vi "SigSyn (G3)-Compute Max Level.vi"(0 "Waveform In":T1, 1 "Destination":string, 5 "Filter":T22 {"Stages"."IIR Filter"."Forward Coefficients" format="%.4f"; "Stages"."IIR Filter"."Reverse Coefficients" format="%.4f"}, 9 "Level":T20, 11 "error in (no error)":errorcluster, 12 "Sampling Rate (Hz)":dbl, 13 "Npts":i32) -> (4 "Waveform Out":T1={"Type"=enum."Tone", "Tone"={"Frequency (kHz)"=0.0, "Phase (cycles)"=0.0, "Random phase"=FALSE}, "Pulse Train"={"Pulse width (us)"=0.0, "Pulse rate (Hz)"=0.0, "Gap (ms)"=0.0, "Polarity"=enum."POS", "PT State"={"Template"=[], "Nperiod"=0, "Index"=0, "Pulse Rate (Hz)"=0.0, "Phase (cycles)"=0.0, "Noff"=0}, "Asynch"=FALSE}, "Noise"={"Properties"={"InvFilt"=FALSE, "Aweight"=FALSE, "Seed"=0, "Tokens"=0, "Brickwall"=FALSE}, "Data"={"TokenNum"=0}}, "File"={"Filename"=path "", "Signal"=[], "Channel"=0, "stream"=FALSE, "offset"=0, "nreps"=0, "loops"=0, "Randomize"=FALSE, "order"=[], "Seed"=0, "Tokens"=0}, "FMSweep"={"Rate (oct/s)"=0.0, "Fmin (Hz)"=0.0, "Fmax (Hz)"=0.0, "Ramp (ms)"=0.0, "Linear"=FALSE}, "Chirp Train"={"Params"={"Fmin (kHz)"=4.0, "Fmax (kHz)"=64.0, "Compensate"=FALSE, "Duration (ms)"=2.0}, "Data"={"WF"=[]}}, "Complex Tone"={"Params"={"F0 (Hz)"=0.0, "Band"={"Flow (Hz)"=0.0, "Fhigh (Hz)"=0.0}, "Phase"=enum."Cosine", "Min F0 (Hz)"=0.0, "Max F0 (Hz)"=0.0, "ContinRandPhase"=FALSE, "Max peak factor"=inf, "Max mod depth"=2.0, "MinHarmNum"=0, "MaxHarmNum"=0, "Level Mode"=enum."per component", "% jitter"=0.0}, "Data"={"Ncomp"=0, "MinHarm"=0, "Phase"=[], "Amplitude"=[], "Npts/frame"=0, "Last F0"=0.0, "Fmin"=0.0, "Fmax"=0.0, "Lslope"=0.0, "randphase"=FALSE, "overall rms"=FALSE, "fmult"=[], "jittered"=FALSE}}, "FM"={"Carrier (kHz)"=0.0, "ModRate (Hz)"=0.0, "Depth (Hz)"=0.0, "Phase (cycles)"=0.0}, "Vowel"={"Freqs"="", "Set level"=enum."Total", "Freq"=[], "weights"=[]}, "Ramp"={"Duration (ms)"=0.0}}, 10 "Level out":T20, 14 "Max Level":dbl, 15 "error out":errorcluster)   [LabVIEW 2020]
uses:
  XControls/Waveform XControls/Waveform (G3)/Waveform Data.ctl
  Waveform VIs/Waveform Enum (V3).ctl
  XControls/Waveform XControls/Tone (G3)/Tone.Properties.ctl
  Waveform VIs/Pulse Train VIs/Pulse Train Params.ctl
  Waveform VIs/Pulse Train VIs/Pulse Polarity.ctl
  Waveform VIs/Pulse Train VIs/PT-Continuous State.ctl
  Waveform VIs/Noise VIs/Noise (G3).ctl
  Waveform VIs/Noise VIs/Noise (G3).Properties.ctl
  Waveform VIs/Noise VIs/Noise (G3).Data.ctl
  Waveform VIs/File VIs/StimFile-Params.ctl
  Waveform VIs/FM Sweep VIs/FM Sweep Params.ctl
  Waveform VIs/Chirp Train VIs/Chirp Train.ctl
  Waveform VIs/Chirp Train VIs/Chirp Train Params.ctl
  Waveform VIs/Complex Tone VIs/CT-Params.ctl
  Waveform VIs/Complex Tone VIs/CT-Phase Enum.ctl
  Waveform VIs/Complex Tone VIs/CT-Runtime Data.ctl
  XControls/Waveform XControls/FM Tone/Data.ctl
  XControls/Waveform XControls/Vowel/Vowel.Properties.ctl
  Waveform VIs/Ramp VIs/Ramp.Properties.ctl
  XControls/Filter (G3)/Filter Data.ctl
  XControls/Filter (G3)/Filter Type.ctl
  Filter VIs/Filter-Bandwidth Units.ctl
  XControls/Level (G3)/Level Data.ctl
  XControls/Level (G3)/Level Units (G3).ctl
  XControls/Waveform XControls/Waveform (G3)/Waveform (G3).xctl
  XControls/Level (G3)/Level (G3).xctl
  XControls/Filter (G3)/Filter (G3).xctl
  XControls/Waveform XControls/Tone (G3)/Tone (G3).xctl
  XControls/Waveform XControls/FM Tone/FM Tone.xctl
  XControls/Waveform XControls/Vowel/Vowel.xctl
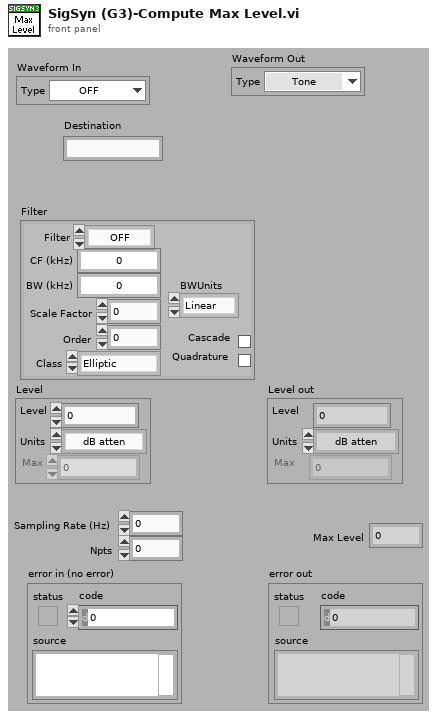
[diagram p1: front panel]
types:
  T1 = typedef "Waveform (G3).xctl/Waveform Data.ctl" = cluster{"Type":T2, "Tone":T3, "Pulse Train":T4, "Noise":T7, "File":T10, "FMSweep":T11, "Chirp Train":T12, "Complex Tone":cluster{"Params":T14, "Data":T16}, "FM":T17, "Vowel":T18, "Ramp":T19}
  T2 = typedef "Waveform Enum (V3).ctl" = enum16{"OFF", "Tone", "Noise", "Pulse Train", "File", "FM Sweep", "Chirp Train", "Complex Tone", "FM Tone", "Vowel", "Ramp"}
  T3 = typedef "Tone (G3).xctl/Tone.Properties.ctl" = cluster{"Frequency (kHz)":dbl, "Phase (cycles)":dbl, "Random phase":bool}
  T4 = typedef "Pulse Train Params.ctl" = cluster{"Pulse width (us)":dbl, "Pulse rate (Hz)":dbl, "Gap (ms)":dbl, "Polarity":T5, "PT State":T6, "Asynch":bool}
  T5 = typedef "Pulse Polarity.ctl" = enum16{"POS", "NEG", "POS-NEG", "NEG-POS"}
  T6 = typedef "PT-Continuous State.ctl" = cluster{"Template":dbl[], "Nperiod":i32, "Index":i32, "Pulse Rate (Hz)":dbl, "Phase (cycles)":dbl, "Noff":i32}
  T7 = typedef "Noise (G3).ctl" = cluster{"Properties":T8, "Data":T9}
  T8 = typedef "Noise (G3).Properties.ctl" = cluster{"InvFilt":bool, "Aweight":bool, "Seed":i32, "Tokens":i32, "Brickwall":bool}
  T9 = typedef "Noise (G3).Data.ctl" = cluster{"TokenNum":i32}
  T10 = typedef "StimFile-Params.ctl" = cluster{"Filename":path, "Signal":dbl[], "Channel":i32, "stream":bool, "offset":i32, "nreps":i32, "loops":i32, "Randomize":bool, "order":i32[], "Seed":i32, "Tokens":i32}
  T11 = typedef "FM Sweep Params.ctl" = cluster{"Rate (oct/s)":dbl, "Fmin (Hz)":dbl, "Fmax (Hz)":dbl, "Ramp (ms)":dbl, "Linear":bool}
  T12 = typedef "Chirp Train.ctl" = cluster{"Params":T13, "Data":cluster{"WF":dbl[]}}
  T13 = typedef "Chirp Train Params.ctl" = cluster{"Fmin (kHz)":dbl, "Fmax (kHz)":dbl, "Compensate":bool, "Duration (ms)":dbl}
  T14 = typedef "CT-Params.ctl" = cluster{"F0 (Hz)":dbl, "Band":cluster{"Flow (Hz)":dbl, "Fhigh (Hz)":dbl}, "Phase":T15, "Min F0 (Hz)":dbl, "Max F0 (Hz)":dbl, "ContinRandPhase":bool, "Max peak factor":dbl, "Max mod depth":dbl, "MinHarmNum":i32, "MaxHarmNum":i32, "Level Mode":enum16{"per component", "overall rms"}, "% jitter":dbl}
  T15 = typedef "CT-Phase Enum.ctl" = enum16{"Cosine", "Random", "Alternating"}
  T16 = typedef "CT-Runtime Data.ctl" = cluster{"Ncomp":i32, "MinHarm":i32, "Phase":dbl[], "Amplitude":dbl[], "Npts/frame":i32, "Last F0":dbl, "Fmin":dbl, "Fmax":dbl, "Lslope":dbl, "randphase":bool, "overall rms":bool, "fmult":dbl[], "jittered":bool}
  T17 = typedef "FM Tone.xctl/Data.ctl" = cluster{"Carrier (kHz)":dbl, "ModRate (Hz)":dbl, "Depth (Hz)":dbl, "Phase (cycles)":dbl}
  T18 = typedef "Vowel.xctl/Vowel.Properties.ctl" = cluster{"Freqs":string, "Set level":enum16{"Total", "Per component"}, "Freq":dbl[], "weights":dbl[]}
  T19 = typedef "Ramp.Properties.ctl" = cluster{"Duration (ms)":dbl}
  T20 = typedef "Level (G3).xctl/Level Data.ctl" = cluster{"Level":dbl, "Units":T21, "Max":dbl, "Data":cluster{"Multiplier":dbl, "Cal File":path, "Cal":cluster{"Freq (Hz)":dbl[], "Mag (dB SPL)":dbl[], "Phase (deg)":dbl[]}, "audiogram":path}}
  T21 = typedef "Level (G3).xctl/Level Units (G3).ctl" = enum16{"dB atten", "dB SPL", "dB re 1 Vrms", "dB V/Hz½", "mW", "dB HL", "Volts", "dB mW"}
  T22 = typedef "Filter (G3).xctl/Filter Data.ctl" = cluster{"Type":T23, "CF (kHz)":dbl, "BW (kHz)":dbl, "Cascade":bool, "Quadrature":bool, "Scale Factor":dbl, "Stages":cluster{"IIR Filter":cluster{"filter structure":enum32{"IIR 2nd Order", "IIR 4th Order"}, "Reverse Coefficients":dbl[], "Forward Coefficients":dbl[]}, "State":dbl[]}[], "Class":enum16{"Elliptic", "Butterworth"}, "Order":i32, "BWUnits":T24}
  T23 = typedef "Filter (G3).xctl/Filter Type.ctl" = enum16{"OFF", "Lowpass", "Highpass", "Bandpass", "Bandstop"}
  T24 = typedef "Filter-Bandwidth Units.ctl" = enum16{"Linear", "Octaves", "Min-Max"}
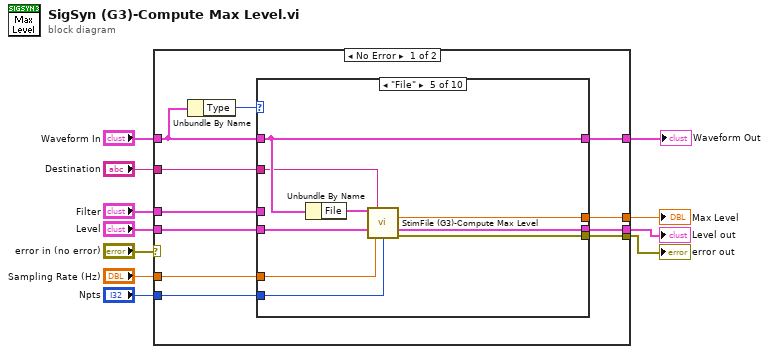
[diagram p0: block diagram]
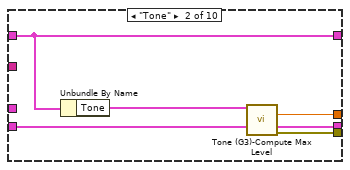
[diagram p3: hidden frame]
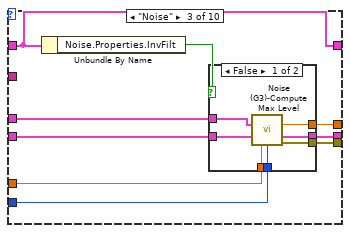
[diagram p4: hidden frame]
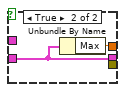
[diagram p5: hidden frame]
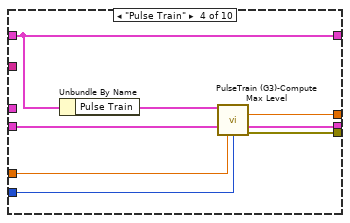
[diagram p6: hidden frame]
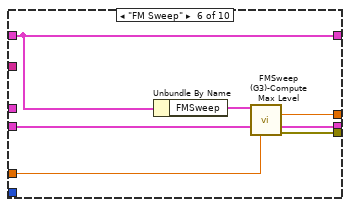
[diagram p7: hidden frame]
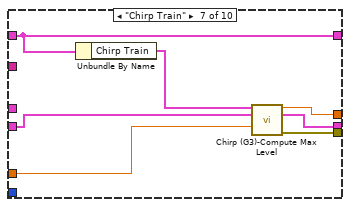
[diagram p8: hidden frame]
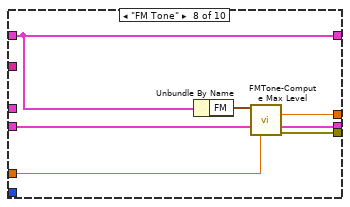
[diagram p9: hidden frame]
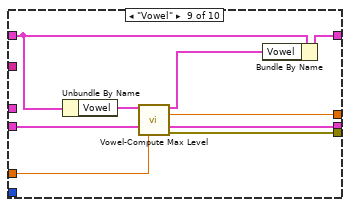
[diagram p10: hidden frame]
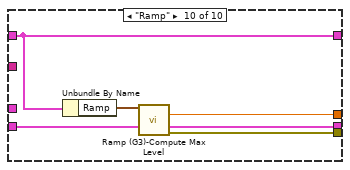
[diagram p11: hidden frame]
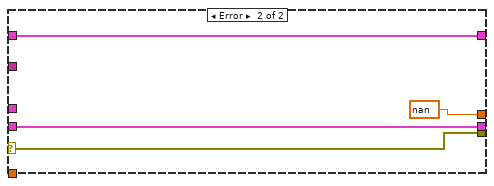
[diagram p12: hidden frame]
diagram:
  n1 = case shown="No Error" "error in (no error)" {
    selector: "error in (no error)" -> [_ w105]
    tunnel: "Level" -> [w20 w103]
    tunnel: "Waveform In" -> [w21 w102]
    tunnel: "Filter" -> [w17 _]
    tunnel: [w15 w105] -> w10
    tunnel: "Npts" -> [w18 _]
    tunnel: [w14 nan ("Reference Level")] -> w5
    tunnel: "Sampling Rate (Hz)" -> [w19 _]
    tunnel: [w16 w103] -> w3
    tunnel: [w13 w102] -> w2
    tunnel: "Destination" -> [w12 _]
    frame No Error {
      n2 = Unbundle By Name(w21) -> ("Type"=w22:T2)
      n3 = case shown="\"File\"" w22 {
        tunnel: w21 -> [w23 w25 w33 w56 w65 w72 w79 w86 w95 w101]
        tunnel: w20 -> [w24 w29 w39 w51 w60 w68 w73 w82 w91 w97]
        tunnel: w19 -> [_ _ w38 w50 w59 w66 w74 w80 w90 _]
        tunnel: w18 -> [_ _ w37 w49 w58 _ _ _ _ _]
        tunnel: w17 -> [_ _ w34 _ _ _ _ _ _ _]
        tunnel: [w24 w27 w31 w53 w63 w69 w76 w83 w92 w98] -> w16
        tunnel: [_ w28 w35 w52 w64 w71 w78 w85 w94 w100] -> w15
        tunnel: [_ w26 w36 w54 w62 w70 w77 w84 w93 w99] -> w14
        tunnel: [w23 w25 w33 w56 w65 w72 w79 w86 w88 w101] -> w13
        tunnel: w12 -> [_ _ _ _ w57 _ _ _ _ _]
        frame "OFF", Default {
        }
        frame "Tone" {
          n4 = Unbundle By Name(w25) -> ("Tone"=w30:T3)
          n5 = call "Tone (G3)-Compute Max Level.vi"("Tone.Properties"=w30, "Level"=w29) -> ("Max Level"=w26:dbl, "Level out"=w27:T20, "error out"=w28:errorcluster)  [unwired: 11 in]
        }
        frame "Noise" {
          n6 = Unbundle By Name(w33) -> ("Noise.Properties.InvFilt"=w32:bool)
          n7 = case shown="False" w32 {
            tunnel: w39 -> [w46 w48]
            tunnel: w38 -> [w45 _]
            tunnel: w37 -> [w44 _]
            tunnel: [w43 w47] -> w36
            tunnel: [w40 w48] -> w31
            tunnel: [w42 _] -> w35
            tunnel: w34 -> [w41 _]
            frame False {
              n8 = call "Noise (G3)-Compute Max Level.vi"("Filter"=w41, "Level"=w46, "Sampling Rate (Hz)"=w45, "Npts"=w44) -> ("Max Level"=w43:dbl, "Level out"=w40:T20, "error out"=w42:errorcluster)  [unwired: 9 in]
            }
            frame True {
              n9 = Unbundle By Name(w48) -> ("Max"=w47:dbl)
            }
          }
        }
        frame "Pulse Train" {
          n10 = Unbundle By Name(w56) -> ("Pulse Train"=w55:T4)
          n11 = call "PulseTrain (G3)-Compute Max Level.vi"("Pulse Train Params"=w55, "Level"=w51, "Sampling Rate (Hz)"=w50, "Npts"=w49) -> ("Max Level"=w54:dbl, "Level out"=w53:T20, "error out"=w52:errorcluster)  [unwired: 9 in]
        }
        frame "File" {
          n12 = Unbundle By Name(w65) -> ("File"=w61:T10)
          n13 = call "StimFile (G3)-Compute Max Level.vi"("File"=w61, "Destination"=w57, "Level"=w60, "Sampling Rate (Hz)"=w59, "Npts"=w58) -> ("Max Level"=w62:dbl, "Level out"=w63:T20, "error out"=w64:errorcluster)  [unwired: 8 in]
        }
        frame "FM Sweep" {
          n14 = Unbundle By Name(w72) -> ("FMSweep"=w67:T11)
          n15 = call "FMSweep (G3)-Compute Max Level.vi"("FMSweep"=w67, "Level"=w68, "Fs (Hz)"=w66) -> ("Max Level"=w70:dbl, "Level out"=w69:T20, "error out"=w71:errorcluster)  [unwired: 10 in]
        }
        frame "Chirp Train" {
          n16 = Unbundle By Name(w79) -> ("Chirp Train"=w75:T12)
          n17 = call "Chirp (G3)-Compute Max Level.vi"("Chirp Train"=w75, "Level in"=w73, "Sampling Rate (Hz)"=w74) -> ("Numeric"=w77:dbl, "Level out"=w76:T20, "error out"=w78:errorcluster)  [unwired: 10 in]
        }
        frame "FM Tone" {
          n18 = Unbundle By Name(w86) -> ("FM"=w81:T17)
          n19 = call "FMTone-Compute Max Level.vi"("FM"=w81, "Level"=w82, "Fs (Hz)"=w80) -> ("Max Level"=w84:dbl, "Level out"=w83:T20, "error out"=w85:errorcluster)  [unwired: 10 in]
        }
        frame "Vowel" {
          n20 = Unbundle By Name(w95) -> ("Vowel"=w89:T18)
          n21 = call "Vowel-Compute Max Level.vi"("Vowel In"=w89, "Level"=w91, "Fs (Hz)"=w90) -> ("Vowel Out"=w87:T18, "Max Level"=w93:dbl, "Level out"=w92:T20, "error out"=w94:errorcluster)  [unwired: 9 in]
          n22 = Bundle By Name(cluster=w95, "Vowel"=w87) -> (w88:T1)
        }
        frame "Ramp" {
          n23 = Unbundle By Name(w101) -> ("Ramp"=w96:T19)
          n24 = call "Ramp (G3)-Compute Max Level.vi"("Ramp.Properties"=w96, "Level"=w97) -> ("Max Level"=w99:dbl, "Level out"=w98:T20, "error out"=w100:errorcluster)  [unwired: 11 in]
        }
      }
    }
    frame Error {
    }
  }
  "error out" <- w10
  "Max Level" <- w5
  "Level out" <- w3
  "Waveform Out" <- w2
